vi "Set Parameter.vi"(8 "error in (no error)":errorcluster, 10 "Parameter":refnum<class "AbstractData.lvclass">, 11 "Stepper3D in":refnum<class "Stepper3D.lvclass">) -> (0 "error out":errorcluster, 3 "Stepper3D out":refnum<class "Stepper3D.lvclass">)   [LabVIEW 2014, in "Stepper3D.lvclass"]
uses:
  Stepper3D.lvclass
  Framework/Model/Data/AbstractData/AbstractData.lvclass
  Framework/Model/Data/DataSingleElement/DataSingleElement.lvclass
  Stepper3D.lvclass/Stepper3D.ctl
  Libs/array.lib/Array.lvlib
  Libs/stepper3D.lib/stepper3D.lvlib
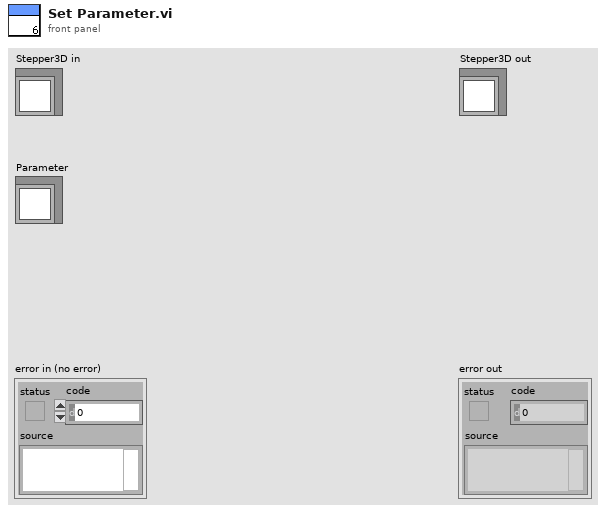
[diagram p1: front panel]
types:
  T1 = typedef "stepper3D.lvlib/CurrentStatus.ctl" = cluster{"desired":dbl[], "current":dbl[], "boundaries":T2[], "is running":bool}
  T2 = typedef "stepper3D.lvlib/BoundaryStatus.ctl" = enum16{"NO BOUNDARY", "OUT OF LEFT", "OUT OF RIGHT"}
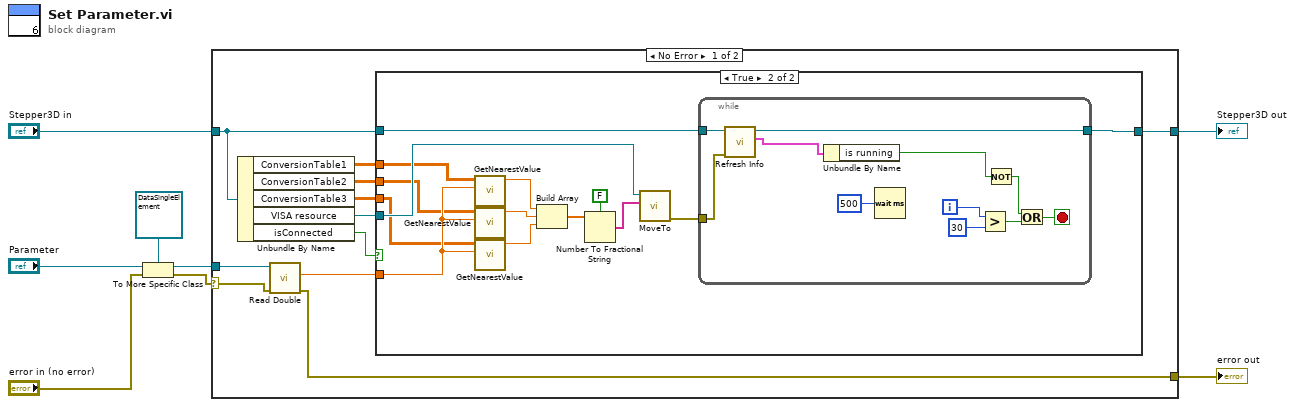
[diagram p0: block diagram]
diagram:
  n1 = To More Specific Class(target class=refnum<class "DataSingleElement.lvclass"> refnum ("DataSingleElement.lvclass"), reference="Parameter", error in="error in (no error)") -> (specific class reference=w8:refnum<class "DataSingleElement.lvclass">, error out=w7:errorcluster)
  n2 = case shown="No Error" w7 {
    selector: w7 -> [w14 w46]
    tunnel: w8 -> [w16 _]
    tunnel: "Stepper3D in" -> [w18 w47]
    tunnel: [w17 w47] -> w1
    tunnel: [w12 w46] -> w4
    frame No Error {
      n3 = Unbundle By Name(w18) -> ("ConversionTable1"=w11:dbl[][], "ConversionTable2"=w10:dbl[][], "ConversionTable3"=w9:dbl[][], "VISA resource"=w19:refnum<visa-resource-name>, "isConnected"=w13:bool)
      n4 = call "Read Double.vi"("error in (no error)"=w14, "DataSingleElement in"=w16) -> ("error out"=w12:errorcluster, "value"=w15:dbl)  [unwired: 7 in, 1 out]
      n5 = case shown="True" w13 {
        tunnel: w19 -> [_ w33]
        tunnel: w18 -> [w20 w29]
        tunnel: [w20 w28] -> w17
        tunnel: w15 -> [_ w34]
        tunnel: w11 -> [_ w26]
        tunnel: w10 -> [_ w25]
        tunnel: w9 -> [_ w24]
        frame False {
        }
        frame True {
          n6 = call "GetNearestValue.vi"("Value"=w34, "Array"=w26) -> ("Nearest Value"=w32:dbl)  [unwired: 9 in]
          n7 = call "GetNearestValue.vi"("Value"=w34, "Array"=w25) -> ("Nearest Value"=w31:dbl)  [unwired: 9 in]
          n8 = call "GetNearestValue.vi"("Value"=w34, "Array"=w24) -> ("Nearest Value"=w30:dbl)  [unwired: 9 in]
          n9 = Build Array(w32, w31, w30) -> (w22:dbl[])
          n10 = Number To Fractional String(use system decimal point (T)=FALSE, number=w22) -> (F-format string=w21:string[])  [unwired: 2 in]
          n11 = call "MoveTo.vi"("positions"=w21, "VISA Refnum in"=w33) -> ("error out"=w27:errorcluster)  [unwired: 8 in, 1 out]
          n12 = while {
            tunnel: w29 -> [w38]
            tunnel: [w35] -> w28
            tunnel: w27 -> [w37]
            i -> [w44]
            stop <- w40 stop-if-true
            n13 = call-dynamic "Refresh Info.vi"("error in (no error)"=w37, "Stepper3D in"=w38) -> ("status"=w36:T1, "Stepper3D out"=w35:refnum<class "Stepper3D.lvclass">)  [unwired: 7 in, 1 out]
            n14 = Unbundle By Name(w36) -> ("is running"=w39:bool)
            n15 = Wait (ms)(milliseconds to wait=u32 500) -> ()  [unwired: 1 out]
            n16 = Greater?(x=w44, y=30) -> (0:w41:bool)
            n17 = Not(x=w39) -> (.not. x?=w42:bool)
            n18 = Or(x=w42, y=w41) -> (x .or. y?=w40:bool)
          }
        }
      }
    }
    frame Error {
    }
  }
  "error out" <- w4
  "Stepper3D out" <- w1
